vi "Settings page.vi"() -> ()   [LabVIEW 2021]
panel:
  out "Global variable Settings":bool
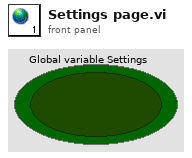
[diagram p1: front panel]
diagram:
